vi "GaGe4_ConfigureAcquisition .vi"(4 "Pre-trigger points":i64, 6 "Total points":i64, 7 "Mode":u16(ring)=1 items=["Single", "Dual", "Quad", "Octal"], 8 "error in (no error)":errorcluster, 9 "Ext. clock":bool, 10 "Sample Rate":dbl, 11 "Handle Cluster in":T1) -> (0 "error out":errorcluster)   [LabVIEW 2015]
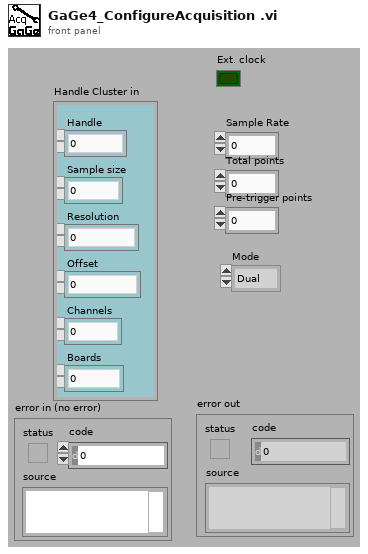
[diagram p1: front panel]
types:
  T1 = cluster{"Handle":u32, "Sample size":u32, "Resolution":i32, "Offset":i32, "Channels":u32, "Boards":u32}
  T2 = cluster{"Sample Rate":dbl, "Clock Mode":enum16{"Internal", "External", "Reference"}, string, dbl, dbl, "Trigger Timeout":dbl, "Trigger Holdoff":dbl, "Trigger Holdoff":dbl}
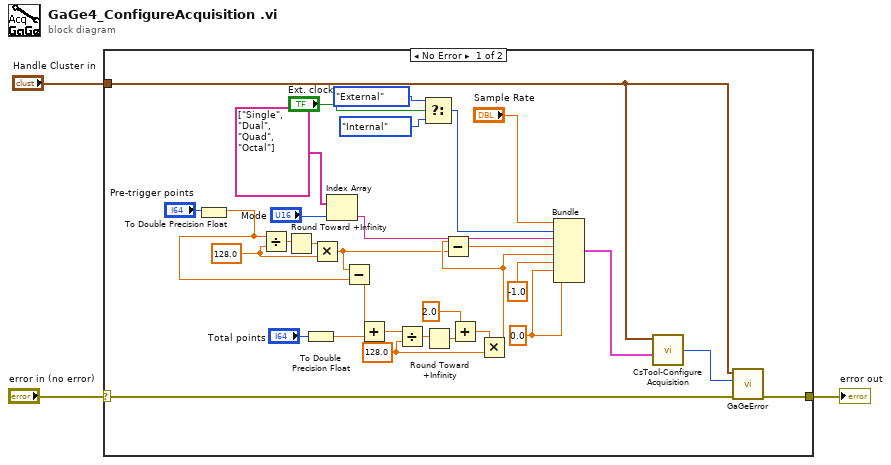
[diagram p0: block diagram]
diagram:
  n1 = case shown="No Error" "error in (no error)" {
    selector: "error in (no error)" -> [w35 w36]
    tunnel: [w34 w36] -> w2
    tunnel: "Handle Cluster in" -> [w33 _]
    frame No Error {
      w15 = 128.0 ("y")
      w16 = 128.0 ("y")
      w22 = 0.0 ("Trigger Holdoff")
      n2 = To Double Precision Float(number="Pre-trigger points") -> (double precision float=w12:dbl)
      n3 = Divide(x=w12, y=w16) -> (x/y=w18:dbl)
      n4 = Round Toward +Infinity(x=w18) -> (ceil(x): smallest int >= x=w17:dbl)
      n5 = To Double Precision Float(number="Total points") -> (double precision float=w20:dbl)
      n6 = Multiply(x=w17, y=w16) -> (x*y=w7:dbl)
      n7 = Index Array(array=string[] ["Single", "Dual", "Quad", "Octal"] ("Strings []"), index="Mode") -> (element=w30:string)
      n8 = Subtract(x=w7, y=w12) -> (x-y=w8:dbl)
      n9 = Add(x=w8, y=w20) -> (x+y=w9:dbl)
      n10 = Divide(x=w9, y=w15) -> (x/y=w19:dbl)
      n11 = Select(t=enum16{"Internal", "External", "Reference"}."External" ("Clock Mode"), s="Ext. clock", f=enum16{"Internal", "External", "Reference"}."Internal" ("Clock Mode")) -> (s? t:f=w25:enum16{"Internal", "External", "Reference"})
      n12 = Round Toward +Infinity(x=w19) -> (ceil(x): smallest int >= x=w6:dbl)
      n13 = Add(x=2.0, y=w6) -> (x+y=w5:dbl)
      n14 = Multiply(x=w5, y=w15) -> (x*y=w10:dbl)
      n15 = Subtract(x=w10, y=w7) -> (x-y=w13:dbl)
      n16 = Bundle("Sample Rate"="Sample Rate", "Clock Mode"=w25, w30, w13, w10, "Trigger Timeout"=-1.0, "Trigger Holdoff"=w22, "Trigger Holdoff"=w22) -> (w23:T2)  [unwired: 1 out]
      n17 = call "CsTool-ConfigureAcquisition.vi"("Handle Cluster"=w33, "Acquisition"=w23) -> ("Error Code"=w32:i32)  [unwired: 3 in]
      n18 = call "GaGeError.vi"("error in (no error)"=w35, "Error Code"=w32, "Handle Cluster"=w33) -> ("error out"=w34:errorcluster)  [unwired: 3 in, 5 out]
    }
    frame Error {
    }
  }
  "error out" <- w2
